vi "ChkSmplDepth.vi"(8 "错误输入（无错误）":errorcluster, 10 "需要设置的采样深度":u16, 11 "当前通道序号":u8) -> (0 "错误输出":errorcluster, 3 "返回值":i32)   [LabVIEW 2014]
uses:
  X86Dll/ZXUTConfigMgr.dll
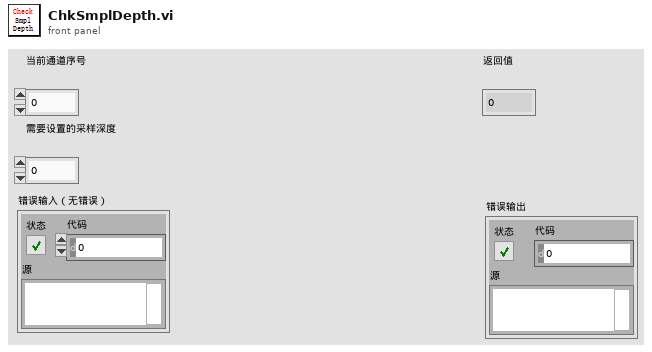
[diagram p1: front panel]
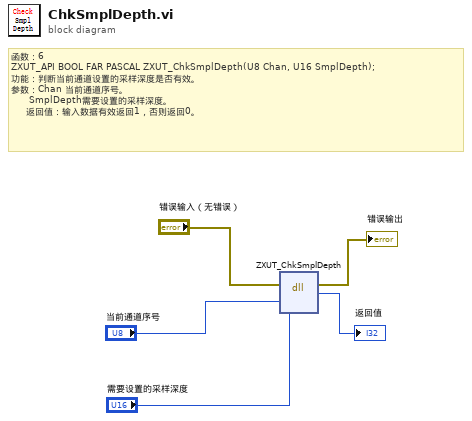
[diagram p0: block diagram]
diagram:
  # "函数：6\nZXUT_API BOOL\tFAR PASCAL ZXUT_ChkSmplDepth(U8 Chan, U16 SmplDepth);\n功能：判断当前通道设置的采样深度是否有效。\n参数：Chan 当前通道序号。\n      SmplDepth需要设置的采样深度。\n\t    返回值：输入数据有效返回1，否则返回0。"
  n1 = dll-call lib="D:/Software/Utrasonic on-line monitoring/X86Dll/ZXUTConfigMgr.dll" fn="ZXUT_ChkSmplDepth"(error in="错误输入（无错误）", "Chan"="当前通道序号", "SmplDepth"="需要设置的采样深度") -> (error out=→"错误输出":errorcluster, "返回值"=→"返回值":i32)  [unwired: 4 in, 1 out]
